vi "Input.vi"(2 "Sign":bool, 3 "Reset":bool, 4 "Dec":T2, 5 "C":bool) -> (0 "Sign":bool, 1 "Bin":T1)   [LabVIEW 2012]
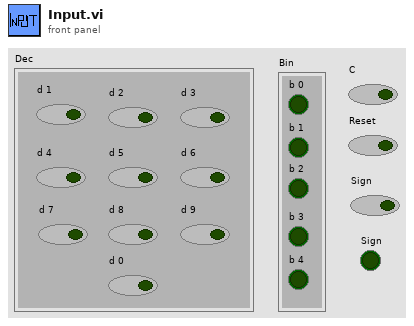
[diagram p1: front panel]
types:
  T1 = cluster{"b 0":bool, "b 1":bool, "b 2":bool, "b 3":bool, "b 4":bool}
  T2 = cluster{"d 0":bool, "d 1":bool, "d 2":bool, "d 3":bool, "d 4":bool, "d 5":bool, "d 6":bool, "d 7":bool, "d 8":bool, "d 9":bool}
  T3 = cluster{"x 0":bool, "x 1":bool, "x 2":bool, "x 3":bool}
  T4 = cluster{"Q 1":bool, "Q 2":bool, "Q 3":bool, "Q 4":bool, "Q 5":bool, "Q 6":bool, "Q 7":bool, "Q 8":bool}
  T5 = cluster{"Q 7":bool, bool, "Q 2":bool, "Q 4":bool, "Q 6":bool, "Q 8":bool}
  T6 = cluster{"X 0":bool, "X 1":bool, "X 2":bool, "X 3":bool, "X 4":bool}
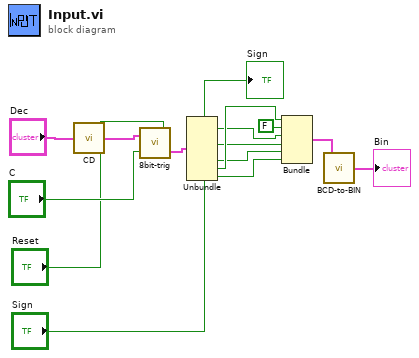
[diagram p0: block diagram]
diagram:
  n1 = call "CD.vi"("dec dig"="Dec") -> ("Bin"=w10:T3)
  n2 = call "8bit-trig.vi"("R"="Reset", "C"="C", "D cluster"=w10) -> ("Cluster Q"=w12:T4)
  n3 = Unbundle(w12) -> ("Q 2"=w1:bool, "Q 4"=w2:bool, "Q 6"=w3:bool, "Q 7"=w5:bool, "Q 8"=w4:bool)  [unwired: 3 out]
  n4 = Bundle("Q 7"=w5, FALSE, "Q 2"=w1, "Q 4"=w2, "Q 6"=w3, "Q 8"=w4) -> (w11:T5)  [unwired: 1 in]
  n5 = call "BCD-to-BIN.vi"("Cluster Y"=w11) -> ("Cluster X"=→"Bin":T6)
  "Sign" <- "Sign"
